vi "pH clear.vi"(3 "index":i32) -> (1 "Buffers":T1(array[cluster]) {"V/T" format="%.2f"; "Buffer" format="%.2f"})   [LabVIEW 2015]
uses:
  DAQ configuration/Sensor buffer command.ctl
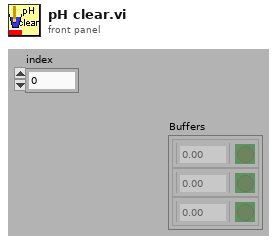
[diagram p1: front panel]
types:
  T1 = cluster{"Buffer":dbl, "Calibrated":bool, "V/T":dbl}[]
  T2 = typedef "Sensor buffer command.ctl" = enum16{"read average", "read recent", "read all", "write", "set buffer size", "Read channel config", "Write channel config", "clear"}
  T3 = typedef "Channel config.ctl" = cluster{"Channel Indices":T4[], "AI Max voltage":dbl[], "Calibration matrix":T5}
  T4 = typedef "channel identifier.ctl" = u16
  T5 = typedef "calib array.ctl" = T6[]
  T6 = typedef "conversion.ctl" = cluster{"conversion matrix":sgl[][], "units":string, "name":string, "scale type":T7, "offset (volts)":dbl, "second channel":i8, "correspondence table":T8, "offset (physical units)":dbl, "pH scale":T9, "D.O.":T10, "Photometer data":T11}
  T7 = typedef "scale type.ctl" = enum16{"Volts", "Polynomial", "Correspondence Table", "pH", "Dissolved Oxygen", "Quadratic", "Photometer"}
  T8 = typedef "correspondence table.ctl" = cluster{"physical units":dbl, "volts":dbl}[]
  T9 = typedef "pH scale.ctl" = cluster{"Buffers":cluster{"Buffer":dbl, "Calibrated":bool, "V/T":dbl}[], "Temperature":dbl}
  T10 = typedef "DO scale.ctl" = cluster{"Temperature":dbl, "K":dbl, "barometric pressure":dbl}
  T11 = typedef "Photometer calibration data.ctl" = cluster{"Dark Voltage":dbl, "Blank Voltage":dbl, "Standards":cluster{"Concentration":dbl, "Voltage":dbl}[]}
  T12 = cluster{"Buffer":dbl, "Calibrated":bool, "V/T":dbl}
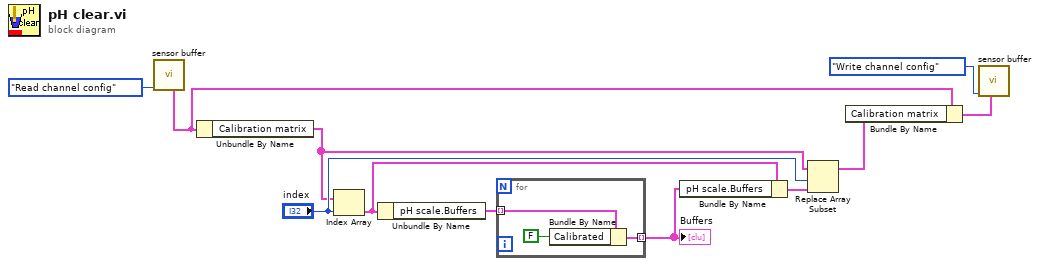
[diagram p0: block diagram]
diagram:
  n1 = call "sensor buffer.vi"("command"=Sensor_buffer_command."Read channel config") -> ("Channel Config out"=w1:T3)  [unwired: 6 in, 4 out]
  n2 = Unbundle By Name(w1) -> ("Calibration matrix"=w5:T5)
  n3 = Index Array(array=w5, index="index") -> (element=w9:T6)
  n4 = Unbundle By Name(w9) -> ("pH scale.Buffers"=w8:T1)
  n5 = for {
    tunnel: w8 -> [w14] mode=indexing
    tunnel: [w13] -> w7 mode=indexing
    n6 = Bundle By Name(cluster=w14, "Calibrated"=FALSE) -> (w13:T12)
  }
  "Buffers" <- w7
  n7 = Bundle By Name(cluster=w9, "pH scale.Buffers"=w7) -> (w11:T6)
  n8 = Replace Array Subset(array=w5, new element=w11, index="index") -> (w3:T5)
  n9 = Bundle By Name(cluster=w1, "Calibration matrix"=w3) -> (w2:T3)
  n10 = call "sensor buffer.vi"("Channel Config"=w2, "command"=Sensor_buffer_command."Write channel config") -> ()  [unwired: 5 in, 5 out]
